vi "construct.vi"(8 "error in (no error)":errorcluster, 9 "configuration name":string, 10 "load config file?":bool=TRUE, 11 "DL090623TwoDAnalyser in":refnum<class "AnalyserDL090623TwoD.lvclass">) -> (0 "error out":errorcluster, 3 "DL090623TwoDAnalyser out":refnum<class "AnalyserDL090623TwoD.lvclass">)   [LabVIEW 2010, in "AnalyserDL090623TwoD.lvclass"]
uses:
  AnalyserDL090623TwoD.lvclass
  AnalyserDL090624Scaffold/AnalyserDL090624Scaffold/AnalyserDL090624Scaffold.lvclass
  AnalyserDL090623TwoD.lvclass/AnalyserDL090623TwoD.ctl
  Segmenter/GenericSegmenter/GenericSegmenter/GenericSegmenter.lvclass
  TraceProcessor/GenericTraceProcessor/GenericTraceProcessor/GenericTraceProcessor.lvclass
  common/classes/ErrorController/ErrorController/class_data.vi
  common/classes/GenericComponent/GenericComponent/GenericComponent.lvclass
  common/classes/ErrorController/ErrorController/ErrorController.lvclass
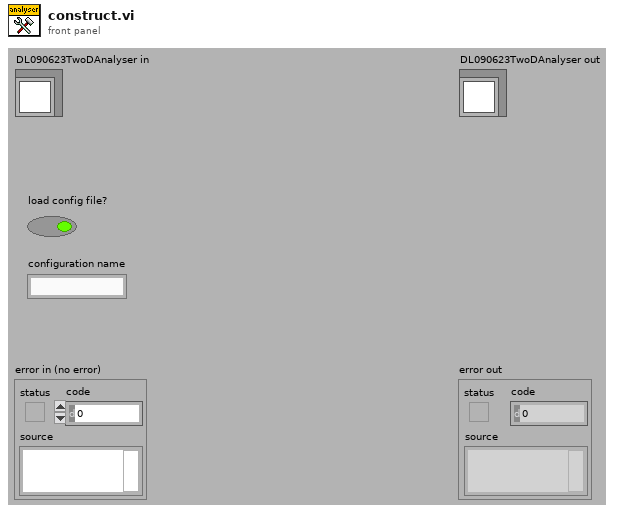
[diagram p1: front panel]
types:
  T1 = typedef "plugin_specification.ctl" = cluster{"class path":string, "configuration":string, "label":string, "settings name":string}
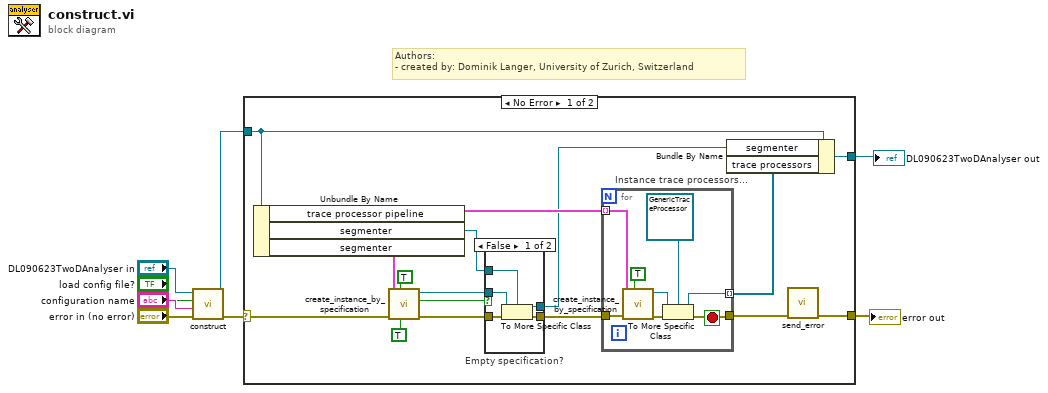
[diagram p0: block diagram]
diagram:
  # "Authors: \n- created by: Dominik Langer, University of Zurich, Switzerland"
  n1 = call-parent "construct.vi"("error in (no error)"="error in (no error)", "configuration name"="configuration name", "load config file?"="load config file?", "GenericPlugin in"="DL090623TwoDAnalyser in") -> ("error out"=w4:errorcluster, "GenericPlugin out"=w3:refnum<class "AnalyserDL090623TwoD.lvclass">)  [unwired: 6 out]
  n2 = case shown="No Error" w4 {
    selector: w4 -> [w20 w40]
    tunnel: w3 -> [w24 w39]
    tunnel: [w12 w40] -> w2
    tunnel: [w23 w39] -> w1
    frame No Error {
      n3 = Unbundle By Name(w24) -> ("trace processor pipeline"=w22:T1[], "segmenter"=w10:refnum<class "GenericSegmenter.lvclass">, "segmenter"=w18:T1)
      n4 = call "create_instance_by_specification.vi"("be tolerant against empty specification?"=TRUE, "call constructor?"=TRUE, "error in (no error)"=w20, "component specification"=w18) -> ("error out"=w19:errorcluster, "empty specification!"=w9:bool, "GenericPlugin out"=w17:refnum<class "GenericComponent.lvclass">)  [unwired: 5 in]
      n5 = case "Empty specification?" shown="False" w9 {
        tunnel: w19 -> [w29 w30]
        tunnel: w17 -> [w28 _]
        tunnel: [w27 w30] -> w15
        tunnel: [w26 _] -> w14
        tunnel: w10 -> [w25 _]
        frame False {
          n6 = To More Specific Class(target class=w25, reference=w28, error in=w29) -> (specific class reference=w26:refnum<class "GenericSegmenter.lvclass">, error out=w27:errorcluster)
        }
        frame True {
        }
      }
      n7 = for "Instance trace processors..." {
        tunnel: w22 -> [w37] mode=indexing
        tunnel: [w33] -> w21 mode=indexing
        tunnel: w15 -> [w36]
        tunnel: [w31] -> w13
        stop <- w31 stop-if-true
        n8 = call "create_instance_by_specification.vi"("call constructor?"=TRUE, "error in (no error)"=w36, "component specification"=w37) -> ("error out"=w35:errorcluster, "GenericPlugin out"=w34:refnum<class "GenericComponent.lvclass">)  [unwired: 6 in, 1 out]
        n9 = To More Specific Class(target class=refnum<class "GenericTraceProcessor.lvclass"> refnum ("GenericTraceProcessor.lvclass"), reference=w34, error in=w35) -> (specific class reference=w33:refnum<class "GenericTraceProcessor.lvclass">, error out=w31:errorcluster)
      }
      n10 = Bundle By Name(cluster=w24, "segmenter"=w14, "trace processors"=w21) -> (w23:refnum<class "AnalyserDL090623TwoD.lvclass">)
      n11 = call "send_error.vi"("error in (no error)"=w13) -> ("error out"=w12:errorcluster)  [unwired: 10 in]
    }
    frame Error {
    }
  }
  "error out" <- w2
  "DL090623TwoDAnalyser out" <- w1
